vi "API Get Token.vi"(6 "Connect to Legacy?":bool, 8 "error in (no error)":errorcluster, 9 "Existing Token":string, 10 "API Port (80)":u16=80, 11 "API Server (localhost)":string="localhost") -> (0 "error out":errorcluster, 2 "New token retrieved?":bool, 3 "Token":string)   [LabVIEW 2011]
doc: "This VI sends the \"http://../api/connect\" command to the PIM Web Engine (located on the specified \"API Server\" and \"API Port\") and retrieves the API Token for this session. The token is retrieved the first time this VI is brought into memory, and any time the \"Get New Token\" boolean is set TRUE, otherwise the token is retrieved from memory to limit the number of commands sent."
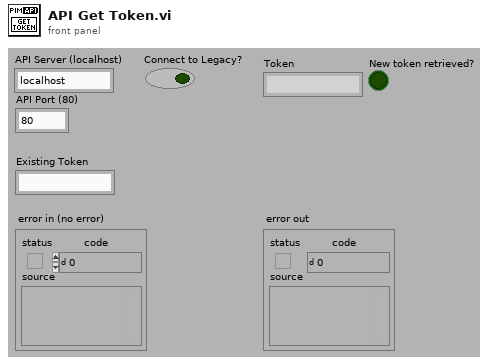
[diagram p1: front panel]
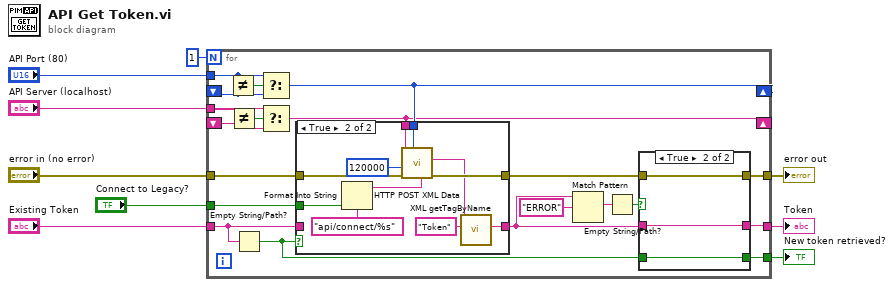
[diagram p0: block diagram]
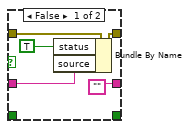
[diagram p2: hidden frame]
diagram:
  n1 = for {
    N: 1 -> [_]
    tunnel: "error in (no error)" -> [w29]
    tunnel: [w24] -> w6
    tunnel: "API Port (80)" -> [w21]
    tunnel: "API Server (localhost)" -> [w16]
    shift-right: [w15] -> _
    shift-left: _ -> [w17]
    shift-right: [w22] -> _
    shift-left: _ -> [w20]
    tunnel: "Existing Token" -> [w14]
    tunnel: [w12] -> w7
    tunnel: "Connect to Legacy?" -> [w13]
    tunnel: [w10] -> w1
    n2 = Not Equal?(x=w21, y=w20) -> (x != y?=w19:bool)
    n3 = Not Equal?(x=w16, y=w17) -> (x != y?=w18:bool)
    n4 = Empty String/Path?(string/path=w14) -> (empty?=w11:bool)
    n5 = Select(t=w21, s=w19, f=w20) -> (s? t:f=w22:u16)
    n6 = Select(t=w16, s=w18, f=w17) -> (s? t:f=w15:string)
    n7 = case shown="True" w11 {
      tunnel: w14 -> [w39 _]
      tunnel: [w39 w46] -> w23
      tunnel: w29 -> [w38 w50]
      tunnel: [w38 w49] -> w27
      tunnel: w22 -> [_ w45]
      tunnel: w15 -> [_ w44]
      tunnel: w13 -> [_ w41]
      frame False {
      }
      frame True {
        n8 = Format Into String(format string="api/connect/%s" ("webService/path (api)"), w41) -> (resulting string=w40:string)  [unwired: 2 in, 1 out]
        n9 = call "HTTP POST XML Data.vi"("webService/path (api)"=w40, "port (80)"=w45, "error in (no error)"=w50, "Timeout ms (30000)"=120000, "address (localhost)"=w44) -> ("error out"=w49:errorcluster, "XML Response"=w48:string)  [unwired: 3 in, 2 out]
        n10 = call "XML getTagByName.vi"("Tag Name"="Token", "XML String"=w48) -> ("Tag Contents"=w46:string)  [unwired: 5 in, 4 out]
      }
    }
    n11 = Match Pattern(string=w23, regular expression="ERROR") -> (match substring=w26:string)  [unwired: 1 in, 3 out]
    n12 = Empty String/Path?(string/path=w26) -> (empty?=w25:bool)
    n13 = case shown="True" w25 {
      tunnel: w27 -> [w34 w37]
      tunnel: [w32 w37] -> w24
      tunnel: w23 -> [w31 w36]
      tunnel: ["" w36] -> w12
      tunnel: w11 -> [_ w35]
      tunnel: [_ w35] -> w10
      frame False {
        n14 = Bundle By Name(cluster=w34, "status"=TRUE, "source"=w31) -> (w32:errorcluster)
      }
      frame True {
      }
    }
  }
  "Token" <- w7
  "error out" <- w6
  "New token retrieved?" <- w1
